vi "Timer.vi"(8 "error in (no error)":errorcluster, 10 "Target Time":dbl=5.0, 11 "Enum":T1(ring)=enum."Get Time") -> (0 "error out":errorcluster, 1 "Paused?":bool, 2 "Time Elapsed?":bool=TRUE, 3 "Elapsed Time":dbl=1653.7379999160767)   [LabVIEW 2024]
doc: "This timer contains start, stop, pause and unpause functionality. It is a functional global variable that stores timing information to help determine when to move between steps."
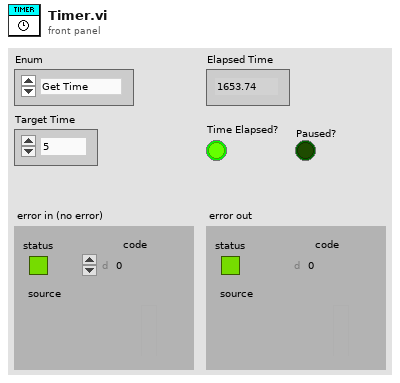
[diagram p1: front panel]
types:
  T1 = enum16{"Start Timer", "Get Time", "Pause", "Unpause"}
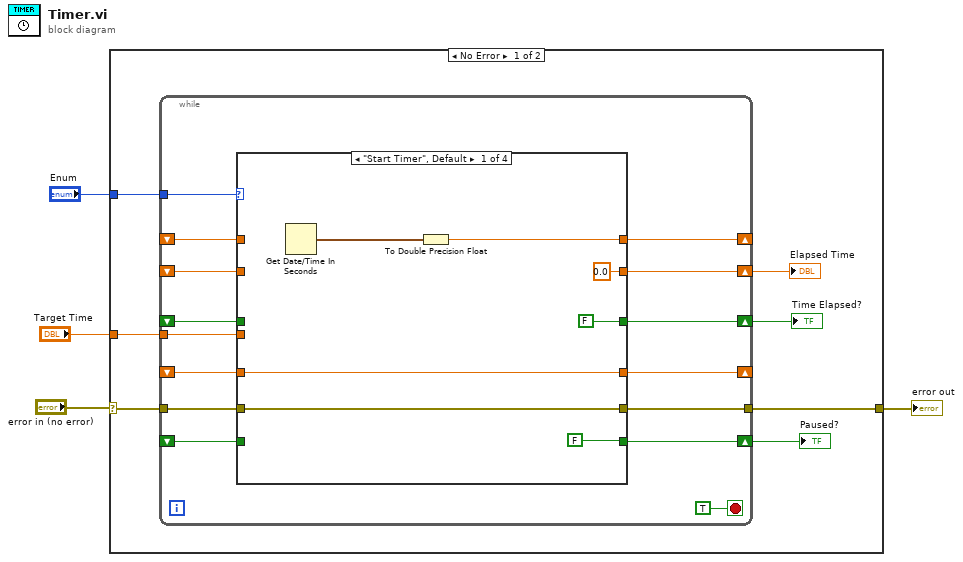
[diagram p0: block diagram]
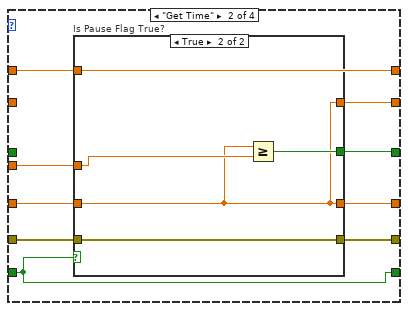
[diagram p2: hidden frame]
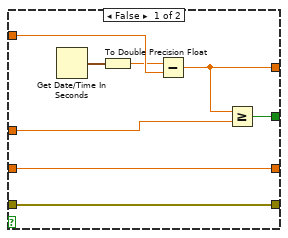
[diagram p3: hidden frame]
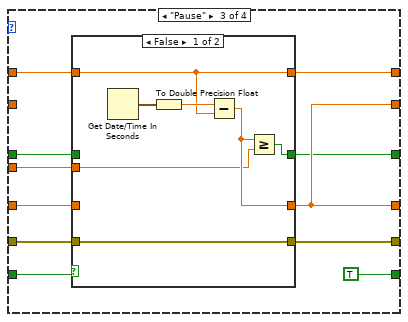
[diagram p4: hidden frame]
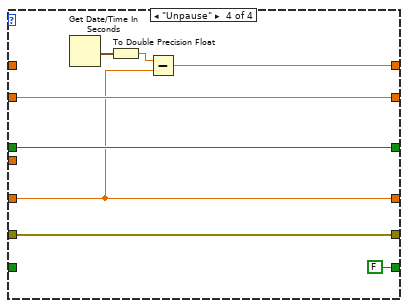
[diagram p6: hidden frame]
diagram:
  n1 = case shown="No Error" "error in (no error)" {
    selector: "error in (no error)" -> [w10 w85]
    tunnel: [w11 w85] -> w3
    tunnel: "Enum" -> [w9 _]
    tunnel: "Target Time" -> [w6 _]
    frame No Error {
      n2 = while {
        tunnel: [w25] -> w11
        tunnel: w10 -> [w24]
        tunnel: w9 -> [w23]
        shift-right: [w22] -> _
        shift-left: _ -> [w21]
        tunnel: w6 -> [w18]
        shift-right: [w17] -> _
        shift-left: _ -> [w14]
        shift-right: [w16] -> w5
        shift-left: _ -> [w15]
        shift-right: [w19] -> w7
        shift-left: _ -> [w13]
        shift-right: [w20] -> w8
        shift-left: _ -> [w12]
        stop <- TRUE stop-if-true
        n3 = case shown="\"Start Timer\", Default" w23 {
          tunnel: [w33 w35 w62 w83] -> w25
          tunnel: w24 -> [w33 w34 w61 w83]
          tunnel: [w29 w42 w58 w80] -> w22
          tunnel: w21 -> [_ w42 w65 _]
          tunnel: [0.0 w41 w63 w79] -> w20
          tunnel: [FALSE w39 w57 w78] -> w19
          tunnel: w18 -> [_ w40 w55 _]
          tunnel: [w27 w36 w63 w77] -> w17
          tunnel: [FALSE w38 TRUE FALSE] -> w16
          tunnel: w15 -> [_ w38 w60 _]
          tunnel: w14 -> [w27 w37 w59 w77]
          tunnel: w13 -> [_ _ w56 w78]
          tunnel: w12 -> [_ _ _ w79]
          frame "Start Timer", Default {
            n4 = Get Date/Time In Seconds() -> (seconds since 1Jan1904=w30:timestamp)
            n5 = To Double Precision Float(number=w30) -> (double precision float=w29:dbl)
          }
          frame "Get Time" {
            n6 = case "Is Pause Flag True?" shown="True" w38 {
              tunnel: w42 -> [w50 _]
              tunnel: [w49 w52] -> w41
              tunnel: w40 -> [w48 w53]
              tunnel: [w47 w54] -> w39
              tunnel: w37 -> [w44 w52]
              tunnel: [w44 w52] -> w36
              tunnel: [w43 w51] -> w35
              tunnel: w34 -> [w43 w51]
              frame False {
                n7 = Get Date/Time In Seconds() -> (seconds since 1Jan1904=w46:timestamp)
                n8 = To Double Precision Float(number=w46) -> (double precision float=w45:dbl)
                n9 = Subtract(x=w45, y=w50) -> (x-y=w49:dbl)
                n10 = Greater Or Equal?(x=w49, y=w48) -> (x >= y?=w47:bool)
              }
              frame True {
                n11 = Greater Or Equal?(x=w52, y=w53) -> (x >= y?=w54:bool)
              }
            }
          }
          frame "Pause" {
            n12 = case shown="False" w60 {
              tunnel: w65 -> [w69 w75]
              tunnel: [w68 w76] -> w63
              tunnel: [w70 w74] -> w62
              tunnel: w61 -> [w70 w74]
              tunnel: w59 -> [_ w76]
              tunnel: [w69 w75] -> w58
              tunnel: [w66 w73] -> w57
              tunnel: w56 -> [_ w73]
              tunnel: w55 -> [w67 _]
              frame False {
                n13 = Get Date/Time In Seconds() -> (seconds since 1Jan1904=w71:timestamp)
                n14 = To Double Precision Float(number=w71) -> (double precision float=w72:dbl)
                n15 = Subtract(x=w72, y=w69) -> (x-y=w68:dbl)
                n16 = Greater Or Equal?(x=w68, y=w67) -> (x >= y?=w66:bool)
              }
              frame True {
              }
            }
          }
          frame "Unpause" {
            n17 = Get Date/Time In Seconds() -> (seconds since 1Jan1904=w81:timestamp)
            n18 = To Double Precision Float(number=w81) -> (double precision float=w82:dbl)
            n19 = Subtract(x=w82, y=w77) -> (x-y=w80:dbl)
          }
        }
      }
      "Elapsed Time" <- w8
      "Time Elapsed?" <- w7
      "Paused?" <- w5
    }
    frame Error {
    }
  }
  "error out" <- w3
